vi "SP Calculate Group Delay.vi"(2 "dF, MHz":dbl, 3 "Phase, radians":dbl[](array[numeric])) -> (1 "Group Delay, seconds":dbl[](array[numeric]))   [LabVIEW 2011]
uses:
  <vilib>/Analysis/NI_AALPro.lvlib
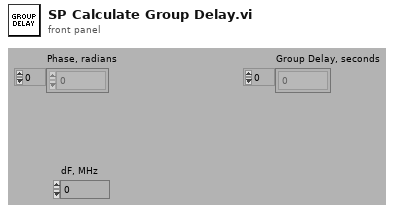
[diagram p1: front panel]
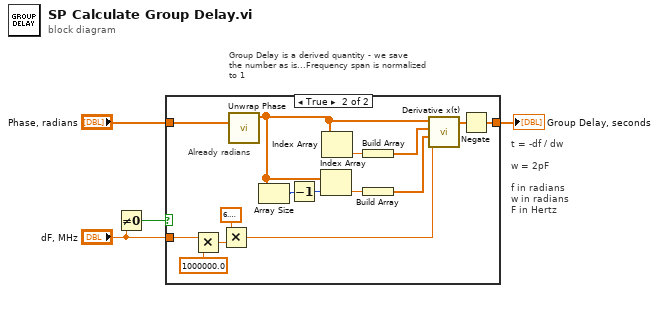
[diagram p0: block diagram]
diagram:
  # "t = -df / dw\n\nw = 2pF\n\nf in radians\nw in radians\nF in Hertz"
  # "Group Delay is a derived quantity - we save \nthe number as is...Frequency span is normalized\nto 1"
  n1 = Not Equal To 0?(x="dF, MHz") -> (x != 0?=w4:bool)
  n2 = case shown="True" w4 {
    tunnel: [w5 w14] -> w2
    tunnel: "Phase, radians" -> [w5 w13]
    tunnel: "dF, MHz" -> [_ w15]
    frame False {
    }
    frame True {
      # "Already radians"
      n3 = Multiply(x=w15, y=1000000.0) -> (x*y=w17:dbl)
      n4 = Multiply(x=6.283185307179586, y=w17) -> (x*y=w16:dbl)
      n5 = call <vilib>:"Unwrap Phase.vi"("Phase"=w13) -> ("Unwrapped Phase"=w10:dbl[])  [unwired: 1 in, 9 out]
      n6 = Array Size(array=w10) -> (size(s)=w11:i32)
      n7 = Decrement(x=w11) -> (x-1=w9:i32)
      n8 = Index Array(array=w10, index=w9) -> (element=w8:dbl)
      n9 = Index Array(array=w10) -> (element=w12:dbl)  [unwired: 1 in]
      n10 = Build Array(w12) -> (w7:dbl[])
      n11 = Build Array(w8) -> (w6:dbl[])
      n12 = call <vilib>:"Derivative x(t).vi"("dt"=w16, "Final Condition"=w6, "Initial Condition"=w7, "X"=w10) -> ("dX/dt"=w20:dbl[])  [unwired: 1 in, 6 out]
      n13 = Negate(x=w20) -> (-x=w14:dbl[])
    }
  }
  "Group Delay, seconds" <- w2
